vi "Line Configuration Dialog.vi"(8 "error in":errorcluster, 9 "engine configuration in":refnum<class "engine configuration.lvclass">, 10 "tag bus configurable plugin module configuration":refnum<class "Multiplexer configuration.lvclass">, 11 "Line":T2) -> (0 "error out":errorcluster, 1 "success":bool, 2 "changed":bool, 3 "Mappings out":T1)   [LabVIEW 2021, in "Multiplexer editor node.lvclass"]
doc: "A dialog for allowing a user to specify the values of a new line."
uses:
  Multiplexer editor node.lvclass
  configuration/Line.ctl
  <vilib>/NI/Tag Bus Module Framework/channel/TBM channel.lvclass
  C:/Program Files (x86)/National Instruments/LabVIEW 2021/vi.lib/NI/Tag Bus/tag/tag descriptor.lvclass
  Mappings.ctl
  Map.ctl
  <vilib>/NI/Module Execution Interface/Engine Configuration/engine configuration.lvclass
  configuration/Multiplexer configuration.lvclass
  C:/Program Files (x86)/National Instruments/LabVIEW 2021/vi.lib/NI/Configuration Framework/serializable configuration/NISE_CEF_serializable configuration.lvclass
  <vilib>/NI/Configuration Framework/serializable configuration/NISE_CEF_serializable configuration.lvclass/NISE_CEF_serializable configuration.ctl
  <vilib>/NI/Tag Bus/tag/tag descriptor.lvclass/tag descriptor.ctl
  <vilib>/NI/Tag Bus/tag/write tag name.vi
  <vilib>/NI/Configuration Framework/serializable configuration/Read UID.vi
  <vilib>/Utility/LVClass/Get LV Class Name.vi
  <vilib>/NI/Configuration Framework/error generator/NISE_error generator.vi
  <vilib>/NI/Tag Bus/tag/tag descriptor.lvclass
  <vilib>/NI/DCAF UI Toolkit/Controls/DCAF UI Elements.lvlib
panel:
  in  "Name":string
  in  "Output":u16(ring)
  in  "Select":u16(ring)
  in  "B":u16(ring)
  in  "A":u16(ring)
  out "errors":string
  in  "cancel":bool
  in  "ok":bool
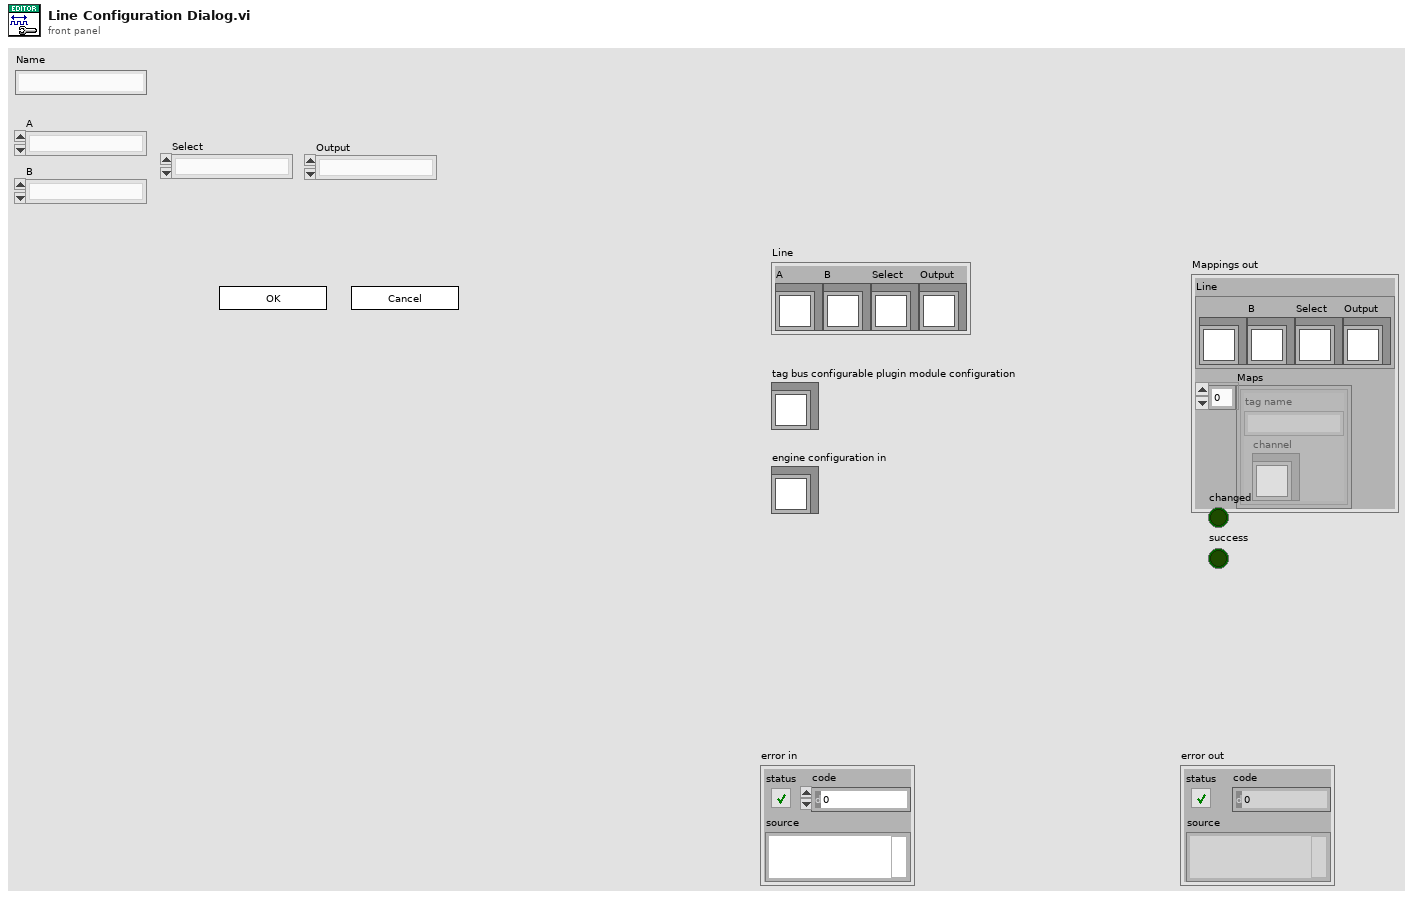
[diagram p1: front panel]
types:
  T1 = typedef "Multiplexer editor node.lvclass/Mappings.ctl" = cluster{"Line":T2, "Maps":T3[]}
  T2 = typedef "Multiplexer configuration.lvclass/Line.ctl" = cluster{"A":refnum<class "TBM channel.lvclass">, "B":refnum<class "TBM channel.lvclass">, "Select":refnum<class "TBM channel.lvclass">, "Output":refnum<class "TBM channel.lvclass">}
  T3 = typedef "Multiplexer editor node.lvclass/Map.ctl" = cluster{"channel":refnum<class "TBM channel.lvclass">, "tag name":string}
  T4 = enum8{"Enabled", "Disabled", "Disabled and Grayed Out"}
  T5 = cluster{"[0]":refnum<class "TBM channel.lvclass">, "[1]":refnum<class "TBM channel.lvclass">, "[2]":refnum<class "TBM channel.lvclass">, "[3]":refnum<class "TBM channel.lvclass">}
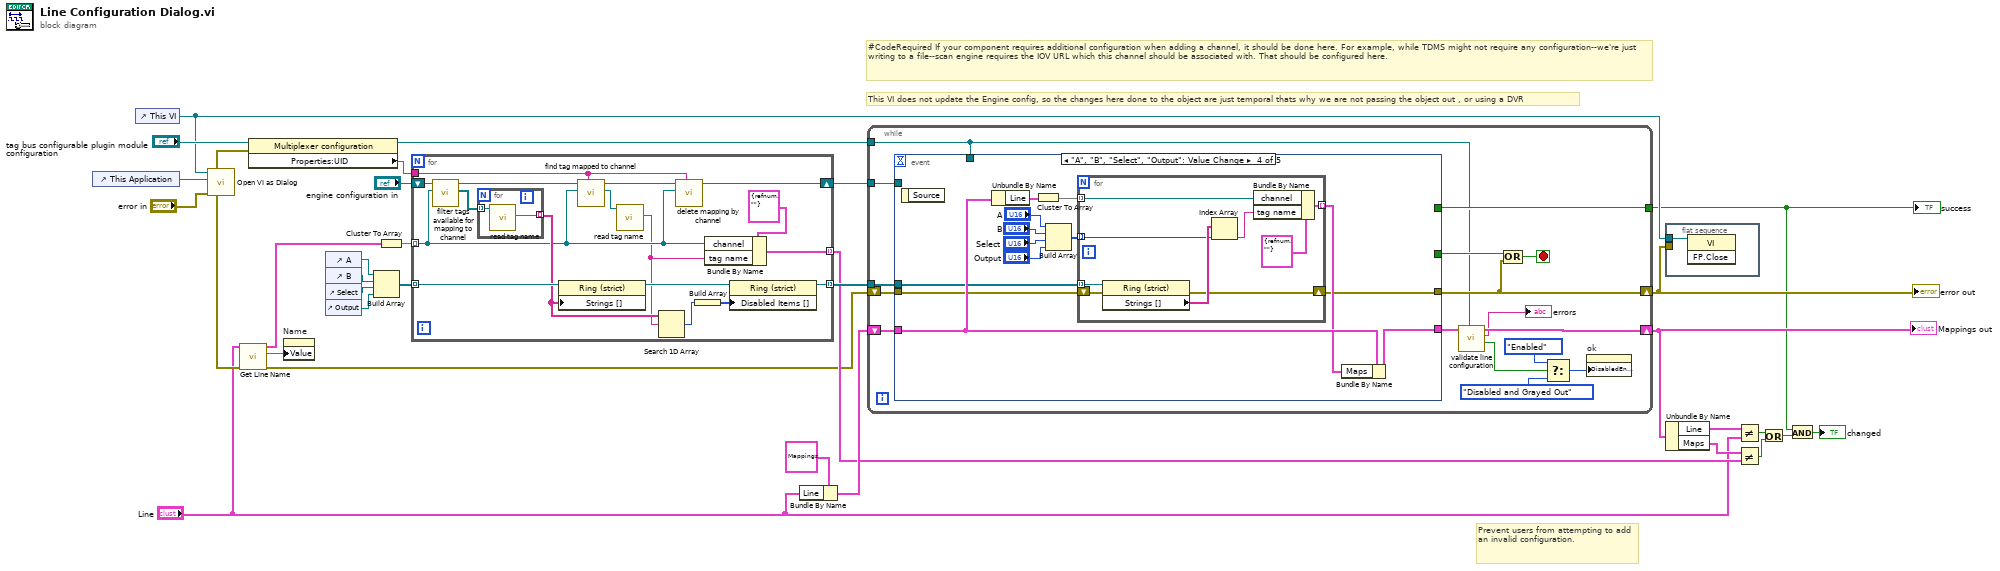
[diagram p0: block diagram]
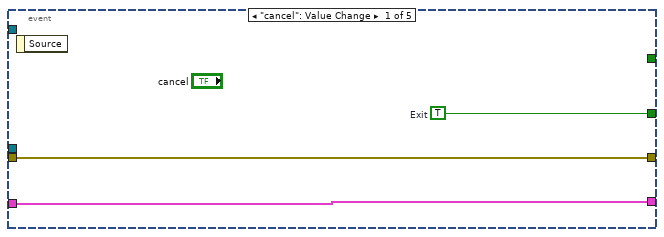
[diagram p2: hidden frame]
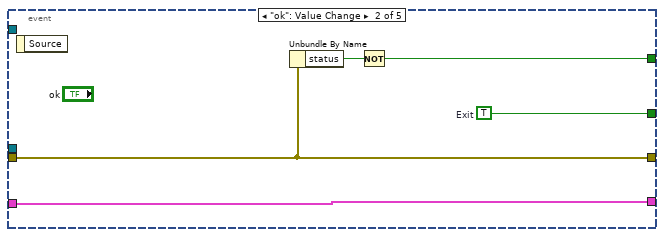
[diagram p3: hidden frame]
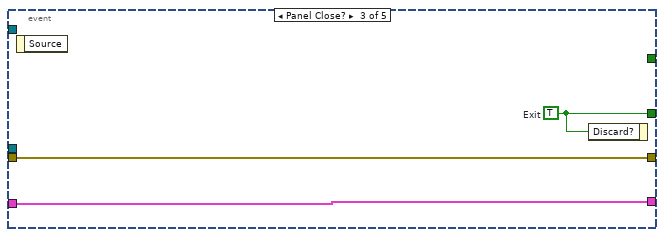
[diagram p4: hidden frame]
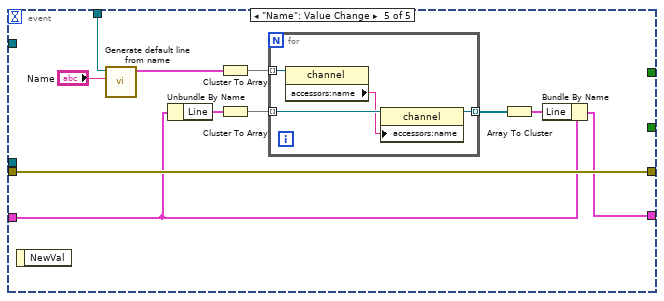
[diagram p5: hidden frame]
diagram:
  # "Prevent users from attempting to add an invalid configuration."
  # "This VI does not update the Engine config, so the changes here done to the object are just temporal thats why we are not passing the object out , or using a DVR"
  # "#CodeRequired If your component requires additional configuration when adding a channel, it should be done here. For example, while TDMS might not require any configuration--we're just writing to a file--scan engine requires the IOV URL which this channel should be associated with. That should be configured here."
  n1 = control-ref of="This Application"() -> (w27:refnum<vi>)
  n2 = control-ref of="This VI"() -> (w22:refnum<vi>)
  n3 = call <vilib>:"Open VI as Dialog.vi"("error in (no error)"="error in", "This Application"=w27, "VI in"=w22) -> ("error out"=w4:errorcluster)  [unwired: 8 in]
  n4 = call "Get Line Name.vi"("error in"=w4, "Line in"="Line") -> ("error out"=w3:errorcluster, "Name"=w5:string, "Line out"=w1:T2)  [unwired: 7 in]
  n5 = property class="Multiplexer configuration"(reference="tag bus configurable plugin module configuration", error in=w4) -> (reference out=w25:refnum<class "Multiplexer configuration.lvclass">, "Properties:UID"=w17:string)  [unwired: 1 out]
  n6 = property on="Name" class="Str"("Value"=w5) -> ()  [unwired: 2 in, 2 out]
  n7 = control-ref of="A"() -> (w13:refnum<vi>)
  n8 = control-ref of="B"() -> (w12:refnum<vi>)
  n9 = control-ref of="Select"() -> (w11:refnum<vi>)
  n10 = control-ref of="Output"() -> (w10:refnum<vi>)
  n11 = Build Array(w13, w12, w11, w10) -> (w9:refnum<vi>[])
  n12 = Cluster To Array(cluster=w1) -> (array=w16:refnum<class "TBM channel.lvclass">[])
  n13 = for {
    tunnel: w17 -> [w38]
    tunnel: w16 -> [w35] mode=indexing
    shift-right: [w49] -> w14
    shift-left: "engine configuration in" -> [w47]
    tunnel: w9 -> [w43] mode=indexing
    tunnel: [w37] -> w8 mode=indexing
    tunnel: [w33] -> w6 mode=indexing
    n14 = call-dynamic "filter tags available for mapping to channel.vi"("channel to map to"=w35, "engine configuration in"=w47) -> ("filtered tags"=w48:refnum<class "tag descriptor.lvclass">[], "engine configuration out"=w46:refnum<class "engine configuration.lvclass">)  [unwired: 8 in]
    n15 = for {
      tunnel: w48 -> [w51] mode=indexing
      tunnel: [w50] -> w42 mode=indexing
      n16 = call <vilib>:"read tag name.vi"("system tag in"=w51) -> ("name"=w50:string)  [unwired: 8 in, 2 out]
    }
    n17 = property class="Ring (strict)"(reference=w43, "Strings []"=w42) -> (reference out=w41:refnum<vi>)  [unwired: 1 in, 1 out]
    n18 = call <vilib>:"find tag mapped to channel.vi"("owner"=w38, "channel"=w35, "engine configuration in"=w46) -> ("tag"=w44:refnum<class "tag descriptor.lvclass">, "engine configuration out"=w45:refnum<class "engine configuration.lvclass">)  [unwired: 6 in, 1 out]
    n19 = call <vilib>:"read tag name.vi"("system tag in"=w44) -> ("name"=w34:string)  [unwired: 8 in, 2 out]
    n20 = Search 1D Array(1D array=w42, element=w34) -> (index of element=w40:i32)  [unwired: 1 in]
    n21 = call <vilib>:"delete mapping by channel.vi"("owner ID"=w38, "channel"=w35, "engine configuration in"=w45) -> ("engine configuration out"=w49:refnum<class "engine configuration.lvclass">)  [unwired: 7 in, 1 out]
    n22 = Build Array(w40) -> (w39:i32[])
    n23 = Bundle By Name(cluster=T3 {"channel"=refnum, "tag name"=""} ("Map"), "channel"=w35, "tag name"=w34) -> (w33:T3)
    n24 = property class="Ring (strict)"(reference=w41, "Disabled Items []"=w39) -> (reference out=w37:refnum<vi>)  [unwired: 1 in, 1 out]
  }
  n25 = Bundle By Name(cluster=T1 {"Line"={"A"=refnum, "B"=refnum, "Select"=refnum, "Output"=refnum}, "Maps"=[]} ("Mappings out"), "Line"="Line") -> (w30:T1)
  n26 = while {
    shift-right: [w59] -> w21
    shift-left: w3 -> [w66]
    tunnel: [w65] -> w20
    shift-right: [w60] -> w28
    shift-left: w30 -> [w62]
    tunnel: w14 -> [w67]
    tunnel: w25 -> [w52]
    tunnel: w8 -> [w53]
    stop <- w63 stop-if-true
    n27 = event shown="[3] \"A\", \"B\", \"Select\", \"Output\": Value Change" {
      selector: _ -> [_ _ _ _ _]
      dyn-events: _ -> [_ _ _ _ _]
      timeout: _ -> [_ _ _ _ _]
      tunnel: w67 -> [_ _ _ _ _]
      tunnel: w66 -> [w70 w73 w78 w80 w111]
      tunnel: [w70 w73 w78 w79 w111] -> w59
      tunnel: [_ w71 _ _ _] -> w65
      tunnel: [w68 w74 w76 _ _] -> w64
      tunnel: w62 -> [w69 w75 w77 w90 w106]
      tunnel: [w69 w75 w77 w91 w107] -> w61
      tunnel: w53 -> [_ _ _ w81 _]
      tunnel: w52 -> [_ _ _ _ w103]
      event "cancel": Value Change {
        w68 = TRUE  # Exit
        n28 = event-data() -> ()  [unwired: 1 in, 1 out]
      }
      event "ok": Value Change {
        w74 = TRUE  # Exit
        n29 = event-data() -> ()  [unwired: 1 in, 1 out]
        n30 = Unbundle By Name(w73) -> ("status"=w72:bool)
        n31 = Not(x=w72) -> (.not. x?=w71:bool)
      }
      event Panel Close? {
        w76 = TRUE  # Exit
        n32 = event-data() -> ()  [unwired: 1 in, 1 out]
        n33 = event-data("Discard?"=w76) -> ()  [unwired: 1 in, 1 out]
      }
      event "A", "B", "Select", "Output": Value Change {
        n34 = event-data() -> ()  [unwired: 1 in, 1 out]
        n35 = Unbundle By Name(w90) -> ("Line"=w89:T2)
        n36 = Cluster To Array(cluster=w89) -> (array=w88:refnum<class "TBM channel.lvclass">[])
        n37 = Build Array("A", "B", "Select", "Output") -> (w82:u16[])
        n38 = for {
          tunnel: w88 -> [w100] mode=indexing
          tunnel: [w99] -> w87 mode=indexing
          tunnel: w82 -> [w95] mode=indexing
          tunnel: w81 -> [w98] mode=indexing
          shift-right: [w92] -> w79
          shift-left: w80 -> [w97]
          n39 = property class="Ring (strict)"(reference=w98, error in=w97) -> (error out=w92:errorcluster, "Strings []"=w96:string[])  [unwired: 1 out]
          n40 = Index Array(array=w96, index=w95) -> (element=w94:string)
          n41 = Bundle By Name(cluster=T3 {"channel"=refnum, "tag name"=""} ("Map"), "channel"=w100, "tag name"=w94) -> (w99:T3)
        }
        n42 = Bundle By Name(cluster=w90, "Maps"=w87) -> (w91:T1)
      }
      event "Name": Value Change {
        n43 = event-data() -> ()  [unwired: 1 in, 1 out]
        n44 = call "Generate default line from name.vi"("Name"="Name", "Multiplexer configuration in"=w103) -> ("Line"=w102:T2)  [unwired: 9 in]
        n45 = Unbundle By Name(w106) -> ("Line"=w110:T2)
        n46 = Cluster To Array(cluster=w102) -> (array=w101:refnum<class "TBM channel.lvclass">[])
        n47 = Cluster To Array(cluster=w110) -> (array=w109:refnum<class "TBM channel.lvclass">[])
        n48 = for {
          tunnel: w109 -> [w114] mode=indexing
          tunnel: [w115] -> w108 mode=indexing
          tunnel: w101 -> [w112] mode=indexing
          n49 = property class="channel"(reference=w112) -> ("accessors:name"=w113:string)  [unwired: 1 in, 2 out]
          n50 = property class="channel"(reference=w114, "accessors:name"=w113) -> (reference out=w115:refnum<class "TBM channel.lvclass">)  [unwired: 1 in, 1 out]
        }
        n51 = Array To Cluster(array=w108) -> (cluster=w105:T5)
        n52 = Bundle By Name(cluster=w106, "Line"=w105) -> (w107:T1)
      }
    }
    n53 = call "validate line configuration.vi"("Module Config"=w52, "Mappings in"=w61) -> ("valid?"=w58:bool, "errors"=→"errors":string, "Mappings out"=w60:T1)  [unwired: 7 in]
    n54 = Compound Arithmetic op=OR(w64, w59) -> (w63:bool)
    n55 = Select(t=T4."Enabled" ("Disabled"), s=w58, f=T4."Disabled and Grayed Out") -> (s? t:f=w55:T4)
    n56 = property on="ok" class="Bool"("DisabledEnum"=w55) -> ()  [unwired: 2 in, 2 out]
  }
  "error out" <- w21
  "success" <- w20
  "Mappings out" <- w28
  n57 = flat-sequence {
    tunnel: w21 -> [_]
    tunnel: w22 -> [w116]
    frame #0 {
      n58 = invoke class="VI" method="FP.Close"(reference=w116) -> ()  [unwired: 2 in, 3 out]
    }
  }
  n59 = Unbundle By Name(w28) -> ("Line"=w29:T2, "Maps"=w7:T3[])
  n60 = Not Equal?(x=w29, y="Line") -> (x != y?=w23:bool)
  n61 = Not Equal?(x=w7, y=w6) -> (x != y?=w24:bool)
  n62 = Or(x=w23, y=w24) -> (x .or. y?=w19:bool)
  n63 = And(x=w20, y=w19) -> (x .and. y?=→"changed":bool)
